vi "Sanitize.vi"(10 "string":string) -> (3 "Sanitized Output":string)   [LabVIEW 2014]
panel:
  out "Sanitize":dbl
  out "Before Sanitize":dbl
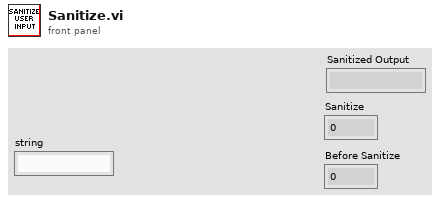
[diagram p1: front panel]
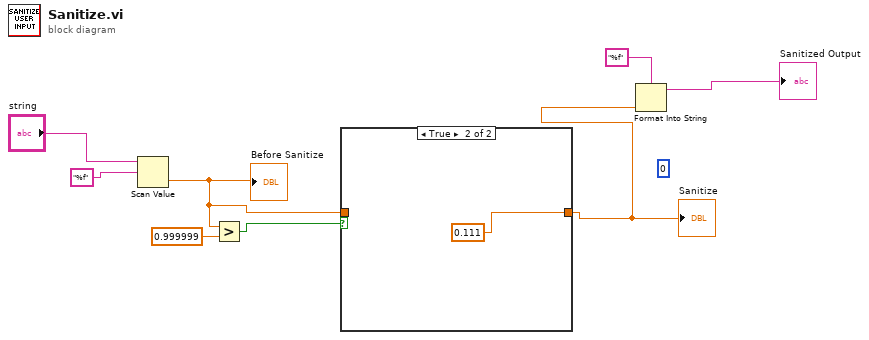
[diagram p0: block diagram]
diagram:
  (unwired) i16 0 ("width (-)")
  n1 = Scan Value(string="string", format string="%f") -> (value=w4:dbl)  [unwired: 1 in, 1 out]
  "Before Sanitize" <- w4
  n2 = Greater?(x=w4, y=0.999999) -> (0:w5:bool)
  n3 = case shown="True" w5 {
    tunnel: w4 -> [w9 _]
    tunnel: [w9 0.111] -> w3
    frame False {
    }
    frame True {
    }
  }
  "Sanitize" <- w3
  n4 = Format Into String(format string="%f", w3) -> (resulting string=→"Sanitized Output":string)  [unwired: 2 in, 1 out]
